vi "Find_Comms.vi"(8 "Fehler (Eingang, kein Fehler)":errorcluster, 11 "serial port name":string="COM3") -> (0 "Fehler (Ausgang)":errorcluster, 1 "VISA-Referenz (Ausgang)":refnum<visa-resource-name>, 2 "Suchergebnisse":string[](array[string]), 3 "serial port name out":string)   [LabVIEW 2020, in "Linearisierung v2.lvlib" / "Gasteiler.lvlib" / "HovaCAL_Interface.lvlib" / "Helper.lvlib"]
uses:
  Helper.lvlib
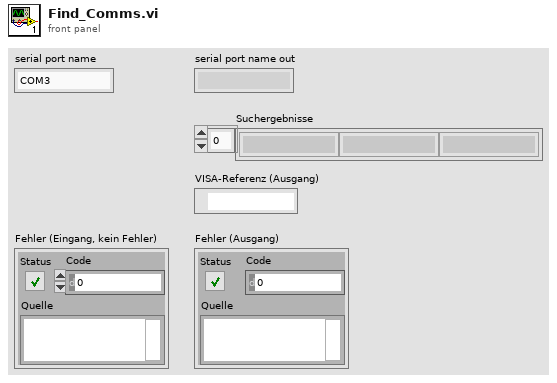
[diagram p1: front panel]
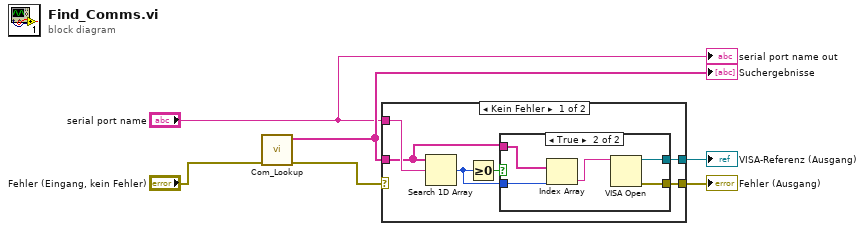
[diagram p0: block diagram]
diagram:
  n1 = call "Com_Lookup.vi"("Fehler (Eingang, kein Fehler)"="Fehler (Eingang, kein Fehler)") -> ("Fehler (Ausgang)"=w2:errorcluster, "find list"=w4:string[])  [unwired: 9 in]
  "Suchergebnisse" <- w4
  n2 = case shown="Kein Fehler" w2 {
    selector: w2 -> [_ w18]
    tunnel: [w12 w18] -> w6
    tunnel: [w11 _] -> w5
    tunnel: w4 -> [w8 _]
    tunnel: "serial port name" -> [w10 _]
    frame No Error {
      n3 = Search 1D Array(1D array=w8, element=w10) -> (index of element=w7:i32)  [unwired: 1 in]
      n4 = Greater Or Equal To 0?(x=w7) -> (x >= 0?=w9:bool)
      n5 = case shown="True" w9 {
        tunnel: [_ w17] -> w12
        tunnel: [_ w16] -> w11
        tunnel: w8 -> [_ w15]
        tunnel: w7 -> [_ w14]
        frame False {
        }
        frame True {
          n6 = Index Array(array=w15, index=w14) -> (element=w13:string)
          n7 = VISA Open(VISA resource name=w13) -> (VISA resource name=w16:refnum<visa-resource-name>, error out=w17:errorcluster)  [unwired: 4 in]
        }
      }
    }
    frame Error {
    }
  }
  "Fehler (Ausgang)" <- w6
  "VISA-Referenz (Ausgang)" <- w5
  "serial port name out" <- "serial port name"
